vi "FTT Sreen.vi"(8 "error in (no error)":errorcluster caption="错误输入（无错误）", 11 "Main":T2={"Tite"="", "Base path"=path "", "Table"=[], "Stations"=[], "Shield Array"=[], "UPHs"=[], "VISA"={"VISA"="", "baud rate"=9600, "data bits"=8, "parity"=enum."None", "stop bits"=10, "flow control"=0}, "Path"={"roof"=path "", "Config"=path "", "Png"=path ""}, "Ctr"={"DB Dispaly"=refnum, "Error Table"=refnum, "Display"=refnum, "Login"=refnum, "Exit"=refnum, "FTT_Submit"=refnum}, "Login"={"User"="", "Grade"=""}, "information"={"cause"="", "Type"=enum."Inform", "code"=0, "Suroce"="", "Status"=FALSE}, "Local DB"={"Connstr"="", "Database"={"Constr"={"Driver"="", "Server"="", "User"="", "Pwd"="", "Database"=""}, "conn ref"=refnum, "State"=FALSE}}, "Remote DB"={"Connstr"="", "Database"={"Constr"={"Driver"="", "Server"="", "User"="", "Pwd"="", "Database"=""}, "conn ref"=refnum, "State"=FALSE}}, "FTT TV"="", "ExchangeTime"=0, "NVH"="", "EOL Path"=path ""} {"VISA"."flow control" items=["None", "XON/XOFF", "RTS/CTS", "XON/XOFF & RTS/CTS", "DTR/DSR", "XON/XOFF & DTR/DSR"]; "VISA"."stop bits" items=["1.0"=10, "1.5"=15, "2.0"=20]}) -> (0 "error out":errorcluster)   [LabVIEW 2014]
uses:
  Type'def/CN Product1_5 Ctr.ctl
  Type'def/CN Product1_4 Ctr.ctl
  Type'def/CN Product Ctr.ctl
  Type'def/Tab.ctl
  Type'def/MainCtr.ctl
  Type'def/UPH Config.ctl
  SubVI's/VISA/Ctr/VISA Ctr.ctl
  Type'def/Main Ctr Ref.ctl
  Type'def/User Login.ctl
  SubVI's/Database/Ctr/Conneect State.ctl
  SubVI's/Database/Ctr/Constr.ctl
  <vilib>/addons/database/Connection.llb/Conn ObjectReference.ctl
  Type'def/CN image Ctr.ctl
  <vilib>/picture/picture.llb/imagedata.ctl
  Type'def/CN Config Ctr.ctl
  <vilib>/addons/database/NI_Database_API.lvlib
panel:
  out "Tab":T1(array[ring])
  out "size(s)":i32
  out "Value":string
  out "Repaired":string
  out "Slash 04":string
  out "End?":bool
  out "Show Tab":T10
  out "Tab CN":enum32{"1/2", "1/3", "1/4", "1/5", "2/5", "3/5"}(tab)
  out "CN image2/2":T11
  out "CN image1/2":T11
  out "CN image3/3":T11
  out "CN image2/3":T11
  out "CN image1/3":T11
  out "CN image4/4":T12
  out "CN image3/4":T12
  out "CN image2/4":T12
  out "CN image1/4":T12
  out "CN image5/5":T13
  out "CN image4/5":T13
  out "CN image3/5":T13
  out "CN image2/5":T13
  out "CN image1/5":T13
  out "CN image5/6":T13
  out "CN image4/6":T13
  out "CN image3/6":T13
  out "CN image2/6":T13
  out "CN image1/6":T13
  out "CN image5/7":T13
  out "CN image4/7":T13
  out "CN image3/7":T13
  out "CN image2/7":T13
  out "CN image1/7":T13
  out "Roof Picture":picture
  out "Vehicle Picture":picture
  out "Line status":string
  out "UPH status":string
  out "Rollo Color status":string
  out "Model":string
  out "Slash 03":string
  out "Slash 01":string
  out "Slash 02":string
  out "FTT Rate":string
  out "Reject":string
  out "Target(%)":string
  out "Target now":string
  out "FTT":string
  out "Actual":string
  out "Plan":string
  out "Repaired and Reject Title":string
  out "Target and Actual Title":string
  out "FTT and FTT Rate Title":string
  out "Plan and Rate Title":string
  out "Error Info 3":string
  out "Error Info 2":string
  out "Error Info":string
  out "Error BG":u32(colorbox)
  out "Time":string
  out "Date":string
  out "Title":string
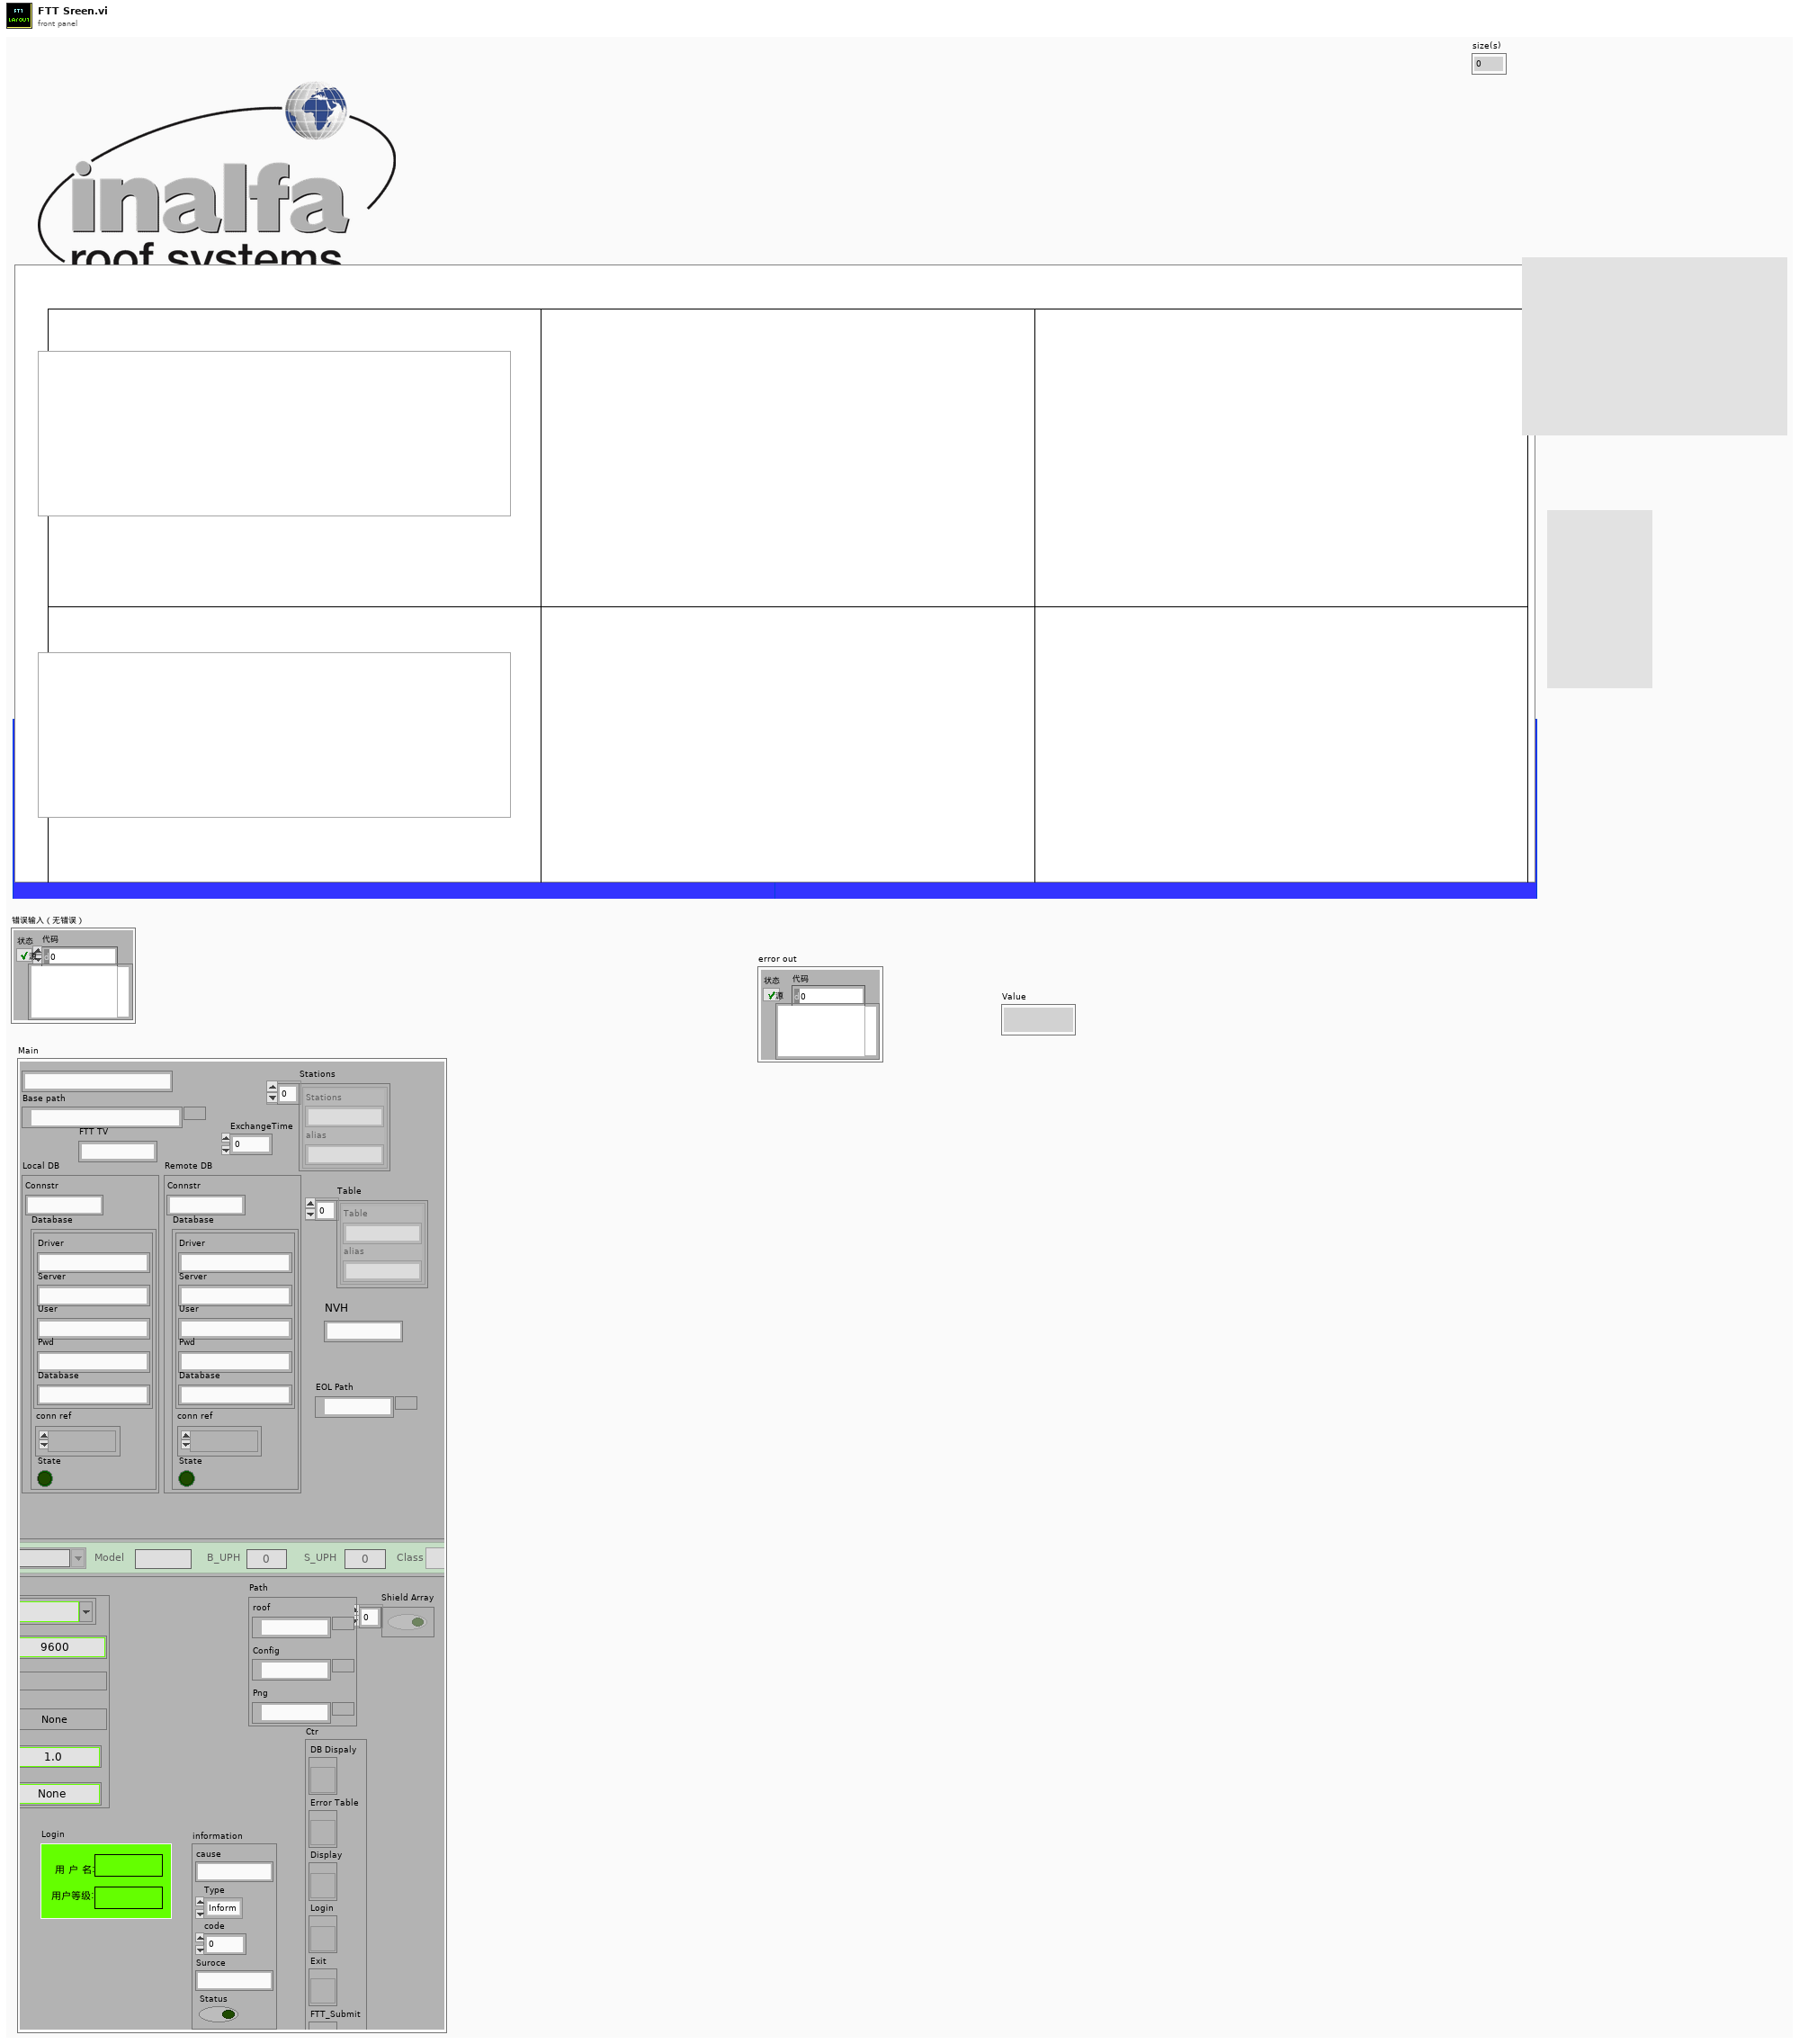
[diagram p1: front panel]
types:
  T1 = enum32{"1/2", "1/3", "1/4", "1/5", "2/5", "3/5"}[]
  T2 = typedef "MainCtr.ctl" = cluster{"Tite":string, "Base path":path, "Table":cluster{"Table":string, "alias":string}[], "Stations":cluster{"Stations":string, "alias":string}[], "Shield Array":bool[], "UPHs":T3[], "VISA":T4, "Path":cluster{"roof":path, "Config":path, "Png":path}, "Ctr":T5, "Login":T6, "information":cluster{"cause":string, "Type":enum16{"Inform", "Warning", "Alarm"}, "code":i32, "Suroce":string, "Status":bool}, "Local DB":cluster{"Connstr":string, "Database":T7}, "Remote DB":cluster{"Connstr":string, "Database":T7}, "FTT TV":string, "ExchangeTime":i32, "NVH":string, "EOL Path":path}
  T3 = typedef "UPH Config.ctl" = cluster{"Line_No":string, "Model":string, "B_UPH ":i16, "S_UPH  ":i16, "Class":enum16{"Big", "Small"}}
  T4 = typedef "VISA Ctr.ctl" = cluster{"VISA":refnum<visa-resource-name>, "baud rate":u32, "data bits":u16, "parity":enum16{"None", "Odd", "Even", "Mark", "Space"}, "stop bits":u16, "flow control":u16}
  T5 = typedef "Main Ctr Ref.ctl" = cluster{"DB Dispaly":refnum<vi>, "Error Table":refnum<vi>, "Display":refnum<vi>, "Login":refnum<vi>, "Exit":refnum<vi>, "FTT_Submit":refnum<vi>}
  T6 = typedef "User Login.ctl" = cluster{"User":string, "Grade":string}
  T7 = typedef "Conneect State.ctl" = cluster{"Constr":T8, "conn ref":T9, "State":bool}
  T8 = typedef "Constr.ctl" = cluster{"Driver":string, "Server":string, "User":string, "Pwd":string, "Database":string}
  T9 = typedef "NI_Database_API.lvlib/Conn ObjectReference.ctl" = refnum<k1>
  T10 = typedef "Tab.ctl" = enum32{"Customer and Shift Info", "Manufacture Info", "Device error info"}
  T11 = typedef "CN Product Ctr.ctl" = cluster{"2D Picture 3":picture, "Model":string, "Brand":string}
  T12 = typedef "CN Product1_4 Ctr.ctl" = cluster{"2D Picture 3":picture, "Model":string, "Brand":string}
  T13 = typedef "CN Product1_5 Ctr.ctl" = cluster{"2D Picture 3":picture, "Model":string, "Brand":string}
  T14 = typedef "imagedata.ctl" = cluster{"image type":i32, "image depth":i32, "image":u8[], "mask":u8[], "colors":u32[], "Rectangle":cluster{"left":i16, "top":i16, "right":i16, "bottom":i16}}
  T15 = cluster{"FTTColor":cluster{"Low":u32, "Middle":u32, "High":u32}, "TargetColor":cluster{"Low":u32, "Middle":u32, "High":u32}}
  T16 = cluster{"FTTRate":cluster{"Low":u32, "High":u32}, "TargetRate":cluster{"Low":u32, "High":u32}}
  T17 = typedef "CN image Ctr.ctl" = cluster{"Images":T14[], "filenames":string[], "Fit Zoom":dbl[], "CN Config":T18[], "CN Enable":T18[], "image Enable":T14[], "CN Ref Enable":refnum<vi>[], "Tab ":enum32{"1/2", "1/3", "1/4", "1/5", "2/5", "3/5"}[], "Pic Enable":refnum<vi>[]}
  T18 = typedef "CN Config Ctr.ctl" = cluster{"Model":string, "Pic_Name":string, "CarName":string, "En/Disable":bool}
  T19 = cluster{"Path":cluster{"roof":path, "Config":path, "Png":path}, "Exit":refnum<vi>, "Show Tab":refnum<vi>, "Target(%)":refnum<vi>, "Repaired":refnum<vi>, "Reject":refnum<vi>, "FTT":refnum<vi>, "FTT Rate":refnum<vi>, "Line status":refnum<vi>, "Vehicle Picture":refnum<vi>, "Roof Picture":refnum<vi>, "Time":refnum<vi>, "Date":refnum<vi>, "Title":refnum<vi>, "Error Info":refnum<vi>, "UPH status":refnum<vi>, "Rollo Color status":refnum<vi>, "Plan":refnum<vi>, "Actual":refnum<vi>, "Repaired":refnum<vi>, "Target now":refnum<vi>, "Range":cluster{"FTTRate":cluster{"Low":u32, "High":u32}, "TargetRate":cluster{"Low":u32, "High":u32}}, "Color":cluster{"FTTColor":cluster{"Low":u32, "Middle":u32, "High":u32}, "TargetColor":cluster{"Low":u32, "Middle":u32, "High":u32}}, "Ctr Color":cluster{"Label":string, "Color":u32}[], "CN Ctr Ref":refnum<vi>[], "CN image":T17, "Tab CN":refnum<vi>}
  T20 = cluster{"seconds":dbl, "Pages":i32, "element":enum32{"1/2", "1/3", "1/4", "1/5", "2/5", "3/5"}}
  T21 = typedef "Main FTT.ctl" = cluster{"Line_Name":string, "Model":string, "Line_State":string, "Color":string, "UPH":string, "Plan":string, "Target Rate":string, "Target":string, "Actual":string, "FTT":string, "FTT Rate":string, "Repaired":string, "Reject":string}
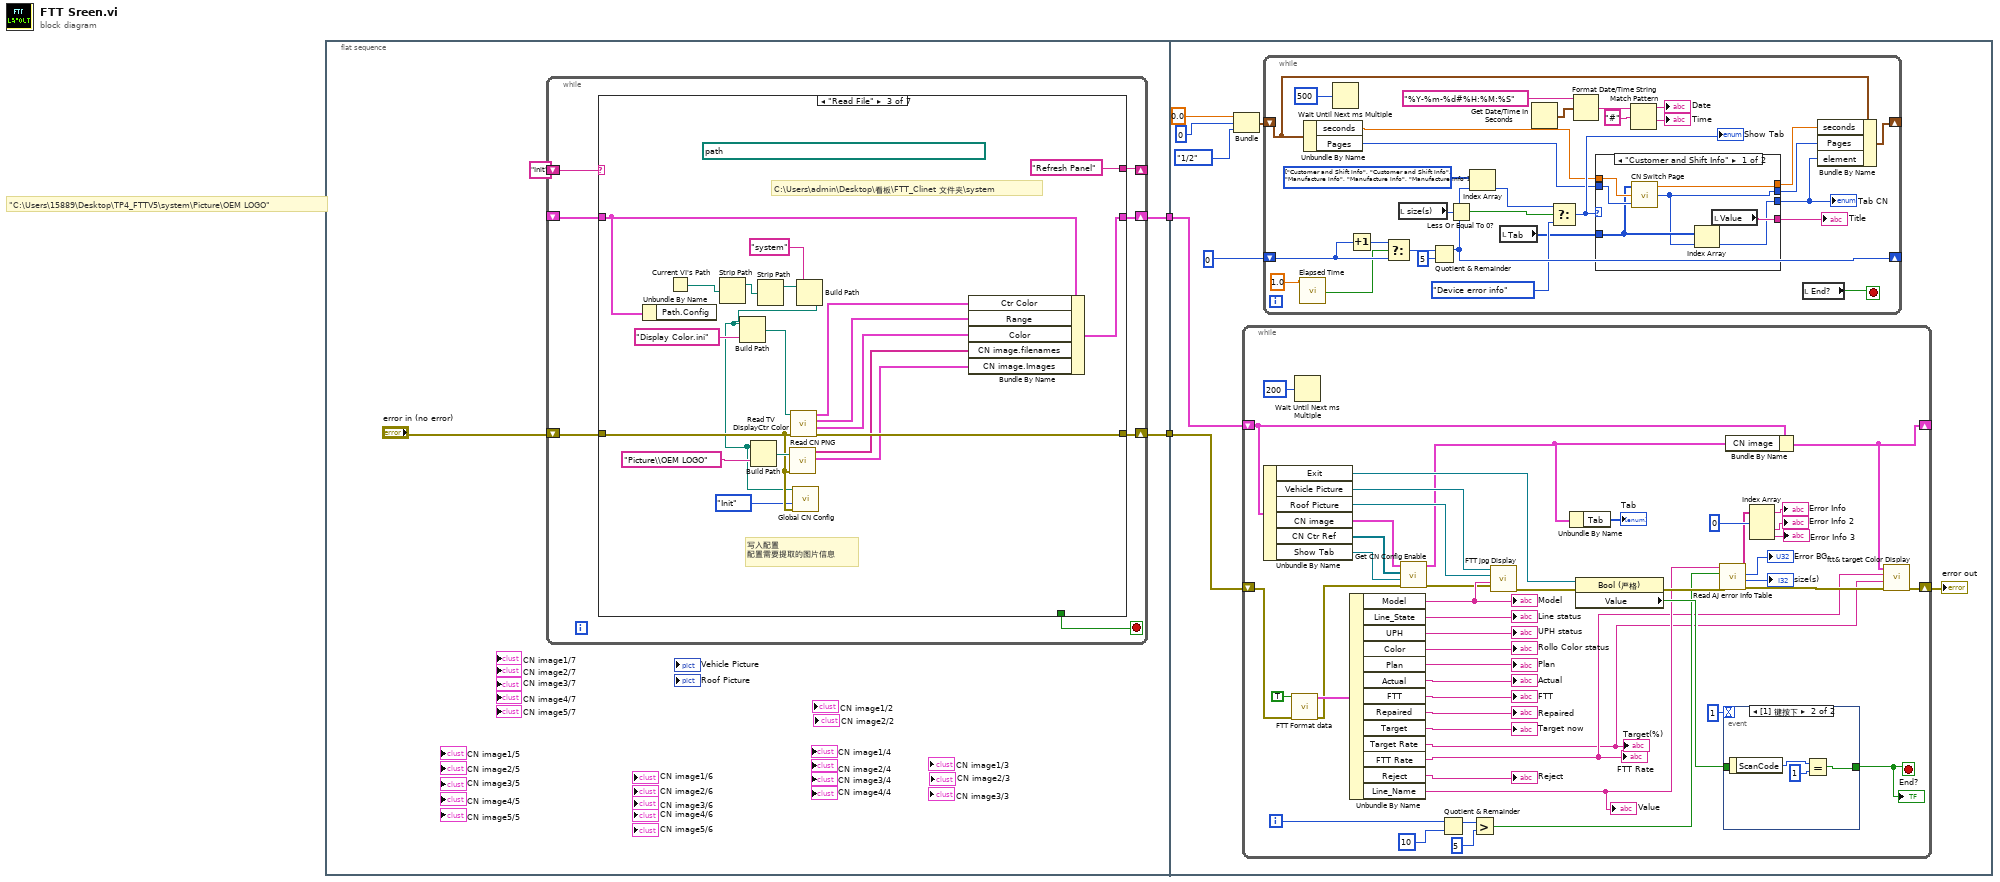
[diagram p0: block diagram]
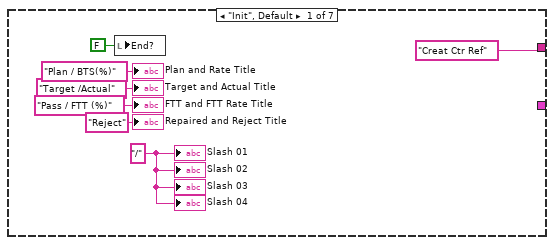
[diagram p2: hidden frame]
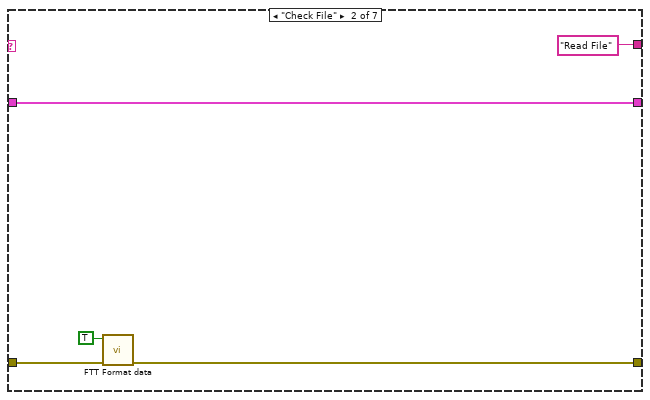
[diagram p3: hidden frame]
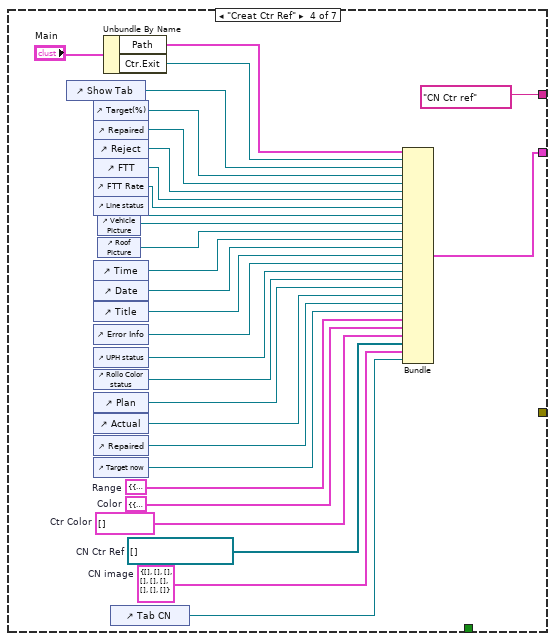
[diagram p4: hidden frame]
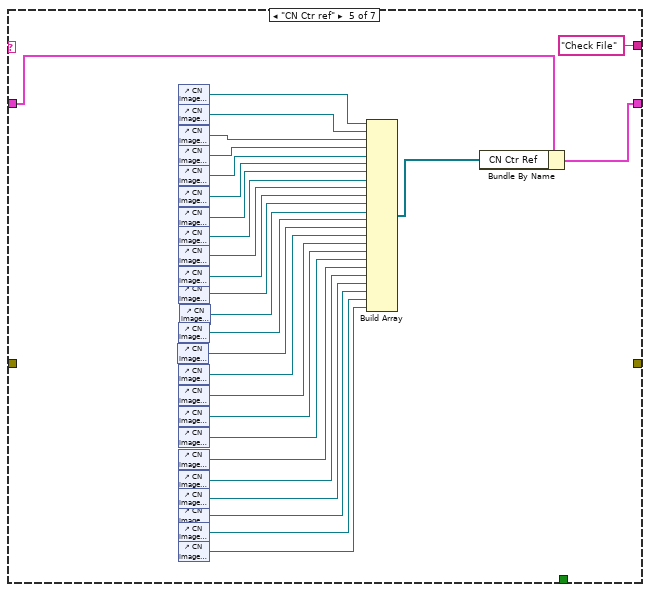
[diagram p5: hidden frame]
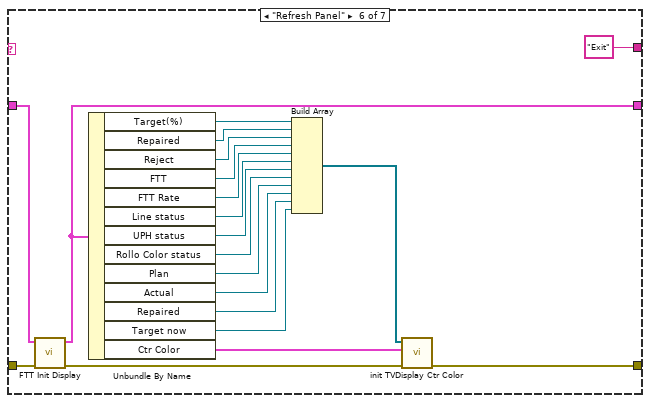
[diagram p6: hidden frame]
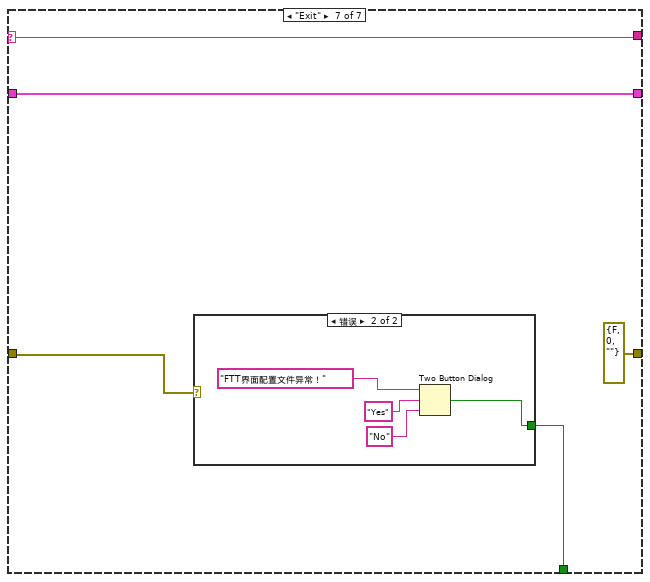
[diagram p7: hidden frame]
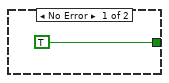
[diagram p8: hidden frame]
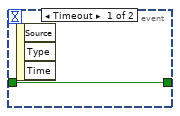
[diagram p9: hidden frame]
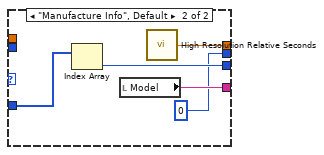
[diagram p10: hidden frame]
diagram:
  # "\"C:\\Users\\15889\\Desktop\\TP4_FTTV5\\system\\Picture\\OEM LOGO\""
  n1 = flat-sequence {
    tunnel: [w4] -> w2
    tunnel: [w3] -> w1
    tunnel: w2 -> [w140]
    tunnel: w1 -> [w141]
    frame #0 {
      n2 = while {
        shift-right: [w12] -> _
        shift-left: "Init" -> [w13]
        shift-right: [w10] -> w3
        shift-left: _ -> [w9]
        shift-right: [w7] -> w4
        shift-left: "error in (no error)" -> [w8]
        stop <- w11 stop-if-true
        n3 = case shown="\"Read File\"" w13 {
          selector: w13 -> [_ _ _ _ _ _ w127]
          tunnel: ["Creat Ctr Ref" "Read File" "Refresh Panel" "CN Ctr ref" "Check File" "Exit" w127] -> w12
          tunnel: [_ _ _ _ _ _ w124] -> w11
          tunnel: [_ w24 w40 w63 w102 w104 w128] -> w10
          tunnel: w9 -> [_ w24 w41 _ w103 w105 w128]
          tunnel: w8 -> [_ w23 w32 _ _ w122 w125]
          tunnel: [_ w22 w42 _ _ w106 errorcluster {"status"=FALSE, "code"=0, "source"=""} ("error out")] -> w7
          frame "Init", Default {
            w16 = "/" ("Slash 01")
            n4 = local write "End?"(FALSE ("End?")) -> ()
            "FTT and FTT Rate Title" <- "Pass / FTT (%)" ("FTT Title")
            "Plan and Rate Title" <- "Plan / BTS(%)" ("Target and Color Title")
            "Target and Actual Title" <- "Target /Actual" ("FTT Title 3")
            "Repaired and Reject Title" <- "Reject" ("FTT Title 4")
            "Slash 02" <- w16
            "Slash 01" <- w16
            "Slash 03" <- w16
            "Slash 04" <- w16
          }
          frame "Check File" {
            n5 = call "FTT Format data.vi"("error in (no error)"=w23, "W/R"=TRUE) -> ("error out"=w22:errorcluster)  [unwired: 6 in, 3 out]
          }
          frame "Read File" {
            (unwired) path "C:/Users/admin/Desktop/V254/FTT Sreen 文件夹/system" ("Path.Config")
            # "写入配置\n配置需要提取的图片信息"
            # "C:\\Users\\admin\\Desktop\\看板\\FTT_Clinet 文件夹\\system"
            n6 = Unbundle By Name(w41) -> ()  [unwired: 1 out]
            n7 = Current VI's Path() -> (path=w30:path)
            n8 = Strip Path(path=w30) -> (stripped path=w29:path)  [unwired: 1 out]
            n9 = Strip Path(path=w29) -> (stripped path=w28:path)  [unwired: 1 out]
            n10 = Build Path(base path=w28, name or relative path="system" ("名称或相对路径")) -> (appended path=w26:path)
            n11 = Build Path(base path=w26, name or relative path="Display Color.ini") -> (appended path=w43:path)
            n12 = Build Path(base path=w26, name or relative path="Picture\\OEM LOGO") -> (appended path=w36:path)
            n13 = call "Read CN PNG.vi"("error in (no error)"=w32, "floder Path"=w36) -> ("Images"=w33:T14[], "filenames"=w34:string[])  [unwired: 7 in, 1 out]
            n14 = call "Read TV DisplayCtr Color.vi"("error in (no error)"=w32, "Path"=w43) -> ("error out"=w42:errorcluster, "Color"=w37:T15, "Range"=w38:T16, "Array"=w39:cluster{"Label":string, "Color":u32}[])  [unwired: 6 in]
            n15 = call "Global CN Config.vi"("error in (no error)"=w32, "Mode"=enum16{"Init", "Read", "Write"}."Init", "Path"=w26) -> ()  [unwired: 7 in, 2 out]
            n16 = Bundle By Name(cluster=w41, "Ctr Color"=w39, "Range"=w38, "Color"=w37, "CN image.filenames"=w34, "CN image.Images"=w33) -> (w40:T19)
          }
          frame "Creat Ctr Ref" {
            w47 = T17 {"Images"=[], "filenames"=[], "Fit Zoom"=[], "CN Config"=[], "CN Enable"=[], "image Enable"=[], "CN Ref Enable"=[], "Tab "=[], "Pic Enable"=[]}  # CN image
            w48 = refnum<vi>[] []  # CN Ctr Ref
            w51 = cluster{"Label":string, "Color":u32}[] []  # Ctr Color
            w52 = T15 {"FTTColor"={"Low"=0, "Middle"=0, "High"=0}, "TargetColor"={"Low"=0, "Middle"=0, "High"=0}}  # Color
            w53 = T16 {"FTTRate"={"Low"=0, "High"=0}, "TargetRate"={"Low"=0, "High"=0}}  # Range
            n17 = control-ref of="Show Tab"() -> (w75:refnum<vi>)
            n18 = control-ref of="Target(%)"() -> (w74:refnum<vi>)
            n19 = control-ref of="Repaired"() -> (w73:refnum<vi>)
            n20 = control-ref of="Reject"() -> (w72:refnum<vi>)
            n21 = control-ref of="FTT"() -> (w71:refnum<vi>)
            n22 = control-ref of="FTT Rate"() -> (w70:refnum<vi>)
            n23 = control-ref of="Line status"() -> (w69:refnum<vi>)
            n24 = control-ref of="Time"() -> (w66:refnum<vi>)
            n25 = control-ref of="Date"() -> (w65:refnum<vi>)
            n26 = control-ref of="Title"() -> (w64:refnum<vi>)
            n27 = control-ref of="Error Info"() -> (w60:refnum<vi>)
            n28 = control-ref of="UPH status"() -> (w59:refnum<vi>)
            n29 = control-ref of="Rollo Color status"() -> (w58:refnum<vi>)
            n30 = control-ref of="Plan"() -> (w57:refnum<vi>)
            n31 = control-ref of="Actual"() -> (w56:refnum<vi>)
            n32 = control-ref of="Repaired"() -> (w55:refnum<vi>)
            n33 = control-ref of="Target now"() -> (w54:refnum<vi>)
            n34 = control-ref of="Vehicle Picture"() -> (w68:refnum<vi>)
            n35 = control-ref of="Roof Picture"() -> (w67:refnum<vi>)
            n36 = Unbundle By Name("Main") -> ("Path"=w49:cluster{"roof":path, "Config":path, "Png":path}, "Ctr.Exit"=w61:refnum<vi>)
            n37 = control-ref of="Tab CN"() -> (w46:refnum<vi>)
            n38 = Bundle("Path"=w49, "Exit"=w61, "Show Tab"=w75, "Target(%)"=w74, "Repaired"=w73, "Reject"=w72, "FTT"=w71, "FTT Rate"=w70, "Line status"=w69, "Vehicle Picture"=w68, "Roof Picture"=w67, "Time"=w66, "Date"=w65, "Title"=w64, "Error Info"=w60, "UPH status"=w59, "Rollo Color status"=w58, "Plan"=w57, "Actual"=w56, "Repaired"=w55, "Target now"=w54, "Range"=w53, "Color"=w52, "Ctr Color"=w51, "CN Ctr Ref"=w48, "CN image"=w47, "Tab CN"=w46) -> (w63:T19)  [unwired: 1 in]
          }
          frame "CN Ctr ref" {
            n39 = control-ref of="CN image5/5"() -> (w88:refnum<vi>)
            n40 = control-ref of="CN image1/2"() -> (w101:refnum<vi>)
            n41 = control-ref of="CN image2/2"() -> (w100:refnum<vi>)
            n42 = control-ref of="CN image1/3"() -> (w99:refnum<vi>)
            n43 = control-ref of="CN image2/3"() -> (w98:refnum<vi>)
            n44 = control-ref of="CN image3/3"() -> (w97:refnum<vi>)
            n45 = control-ref of="CN image1/4"() -> (w96:refnum<vi>)
            n46 = control-ref of="CN image2/4"() -> (w95:refnum<vi>)
            n47 = control-ref of="CN image3/4"() -> (w94:refnum<vi>)
            n48 = control-ref of="CN image4/4"() -> (w93:refnum<vi>)
            n49 = control-ref of="CN image1/5"() -> (w92:refnum<vi>)
            n50 = control-ref of="CN image2/5"() -> (w91:refnum<vi>)
            n51 = control-ref of="CN image4/5"() -> (w89:refnum<vi>)
            n52 = control-ref of="CN image1/6"() -> (w87:refnum<vi>)
            n53 = control-ref of="CN image2/6"() -> (w86:refnum<vi>)
            n54 = control-ref of="CN image3/6"() -> (w85:refnum<vi>)
            n55 = control-ref of="CN image4/6"() -> (w84:refnum<vi>)
            n56 = control-ref of="CN image5/6"() -> (w83:refnum<vi>)
            n57 = control-ref of="CN image1/7"() -> (w82:refnum<vi>)
            n58 = control-ref of="CN image2/7"() -> (w81:refnum<vi>)
            n59 = control-ref of="CN image3/7"() -> (w80:refnum<vi>)
            n60 = control-ref of="CN image4/7"() -> (w79:refnum<vi>)
            n61 = control-ref of="CN image5/7"() -> (w78:refnum<vi>)
            n62 = control-ref of="CN image3/5"() -> (w90:refnum<vi>)
            n63 = Build Array(w101, w100, w99, w98, w97, w96, w95, w94, w93, w92, w91, w90, w89, w88, w87, w86, w85, w84, w83, w82, w81, w80, w79, w78) -> (w77:refnum<vi>[])
            n64 = Bundle By Name(cluster=w103, "CN Ctr Ref"=w77) -> (w102:T19)
          }
          frame "Refresh Panel" {
            n65 = call "FTT Init Display.vi"("error in (no error)"=w122, "Cluster 2"=w105) -> ("error out"=w109:errorcluster, "Cluster out"=w104:T19)  [unwired: 8 in]
            n66 = Unbundle By Name(w104) -> ("Target(%)"=w121:refnum<vi>, "Repaired"=w120:refnum<vi>, "Reject"=w119:refnum<vi>, "FTT"=w118:refnum<vi>, "FTT Rate"=w117:refnum<vi>, "Line status"=w116:refnum<vi>, "UPH status"=w115:refnum<vi>, "Rollo Color status"=w114:refnum<vi>, "Plan"=w113:refnum<vi>, "Actual"=w112:refnum<vi>, "Repaired"=w111:refnum<vi>, "Target now"=w110:refnum<vi>, "Ctr Color"=w107:cluster{"Label":string, "Color":u32}[])
            n67 = Build Array(w121, w120, w119, w118, w117, w116, w115, w114, w113, w112, w111, w110) -> (w108:refnum<vi>[])
            n68 = call "init TVDisplay Ctr Color.vi"("error in (no error)"=w109, "Ctr Color"=w107, "appended array"=w108) -> ("error out"=w106:errorcluster)  [unwired: 8 in]
          }
          frame "Exit" {
            n69 = case shown="错误" w125 {
              tunnel: [TRUE w130] -> w124
              frame No Error {
              }
              frame Error {
                n70 = Two Button Dialog(message="FTT界面配置文件异常！" ("消息"), 1:"No" ("F按钮名称（“取消”）"), 2:"Yes" ("T按钮名称（“确定”）")) -> (T button?=w130:bool)
              }
            }
          }
        }
      }
    }
    frame #1 {
      n71 = Bundle("seconds"=0.0, "Pages"=0, "element"=enum32{"1/2", "1/3", "1/4", "1/5", "2/5", "3/5"}."1/2") -> (w134:T20)  [unwired: 1 in]
      n72 = while {
        shift-right: [w153] -> w139
        shift-left: w140 -> [w181]
        shift-right: [w144] -> _
        shift-left: w141 -> [w147]
        i -> [w167]
        stop <- w169 stop-if-true
        n73 = Unbundle By Name(w147) -> ("Exit"=w171:refnum<vi>, "Vehicle Picture"=w188:refnum<vi>, "Roof Picture"=w187:refnum<vi>, "CN image"=w150:T17, "CN Ctr Ref"=w146:refnum<vi>[], "Show Tab"=w145:refnum<vi>)
        n74 = call "FTT Format data.vi"("error in (no error)"=w181, "W/R"=TRUE) -> ("error out"=w149:errorcluster, "Display"=w186:T21)  [unwired: 6 in, 2 out]
        n75 = Wait Until Next ms Multiple(millisecond multiple=u32 200) -> ()  [unwired: 1 out]
        n76 = Unbundle By Name(w186) -> ("Model"=w184:string, "Line_State"=→"Line status":string, "UPH"=→"UPH status":string, "Color"=→"Rollo Color status":string, "Plan"=→"Plan":string, "Actual"=→"Actual":string, "FTT"=→"FTT":string, "Repaired"=→"Repaired":string, "Target"=→"Target now":string, "Target Rate"=w151:string, "FTT Rate"=w152:string, "Reject"=→"Reject":string, "Line_Name"=w155:string)
        "Model" <- w184
        "Target(%)" <- w151
        "FTT Rate" <- w152
        "Value" <- w155
        n77 = call "Get CN Config Enable.vi"("error in (no error)"=w149, "Show Tab"=w145, "CN Pic Ref"=w146, "CN image"=w150) -> ("error out"=w148:errorcluster, "CN image out"=w143:T17)  [unwired: 6 in]
        n78 = Quotient & Remainder(x=w167, y=10) -> (x-y*floor(x/y)=w165:i32)  [unwired: 1 out]
        n79 = Greater?(x=w165, y=5) -> (0:w163:bool)
        n80 = call "FTT jpg Display.vi"("error in (no error)"=w148, "Model"=w184, "Roof Picture"=w187, "Vehicle Picture"=w188) -> ("错误输出"=w172:errorcluster)  [unwired: 7 in]
        n81 = Unbundle By Name(w143) -> ("Tab"=→"Tab":T1)
        n82 = property class="Bool (严格)"(reference=w171, error in=w172) -> (error out=w168:errorcluster, "Value"=w170:bool)  [unwired: 1 out]
        n83 = call "Read AJ error Info Table.vi"("error in (no error)"=w168, "s"=w163, "Linename"=w155) -> ("error IO"=w154:errorcluster, "size(s)"=→"size(s)":i32, "Error BG"=→"Error BG":u32, "Array"=w156:string[])  [unwired: 5 in]
        n84 = event shown="[1] 键按下" {
          selector: _ -> [_ _]
          dyn-events: _ -> [_ _]
          timeout: 1 -> [_ _]
          tunnel: [w190 w191] -> w169
          tunnel: w170 -> [w190 _]
          event Timeout {
            n85 = event-data() -> ()  [unwired: 1 in, 3 out]
          }
          event Key Down {
            n86 = event-data() -> ("ScanCode"=w193:i16)  [unwired: 1 in]
            n87 = Equal?(x=w193, y=i16 1) -> (x = y?=w191:bool)
          }
        }
        "End?" <- w169
        n88 = Bundle By Name(cluster=w147, "CN image"=w143) -> (w144:T19)
        n89 = Index Array(array=w156, index #1=0 ("index")) -> (element #1=→"Error Info":string, element #2=→"Error Info 2":string, element #3=→"Error Info 3":string)  [unwired: 2 in]
        n90 = call "ftt& target Color Display.vi"("error in (no error)"=w154, "Tatget"=w151, "ftt"=w152, "Cluster"=w144) -> ("error out"=w153:errorcluster)  [unwired: 7 in]
      }
      "error out" <- w139
      n91 = while {
        shift-right: [w212] -> _
        shift-left: u64 0 -> [w221]
        shift-right: [w199] -> _
        shift-left: w134 -> [w200]
        stop <- w208 stop-if-true
        w219 = T10[] [enum."Customer and Shift Info", enum."Customer and Shift Info", enum."Manufacture Info", enum."Manufacture Info", enum."Manufacture Info"] items=["Customer and Shift Info", "Manufacture Info", "Device error info"]
        n92 = call "Elapsed Time"("Time Target (s)"=1.0) -> ("Time has Elapsed"=w207:bool)  [unwired: 11 in, 7 out]
        n93 = Unbundle By Name(w200) -> ("seconds"=w195:dbl, "Pages"=w194:i32)
        n94 = Wait Until Next ms Multiple(millisecond multiple=u32 500) -> ()  [unwired: 1 out]
        n95 = Increment(x=w221) -> (x+1=w220:u64)
        n96 = Select(t=w220, s=w207, f=w221) -> (s? t:f=w214:u64)
        n97 = local read "size(s)"() -> (w203:i32)
        n98 = Quotient & Remainder(x=w214, y=u64 5) -> (x-y*floor(x/y)=w212:u64)  [unwired: 1 out]
        n99 = Less Or Equal To 0?(x=w203) -> (x <= 0?=w202:bool)
        n100 = Index Array(array=w219, index=w212) -> (element=w205:T10)
        n101 = local read "Tab"() -> (w201:T1)
        n102 = Get Date/Time In Seconds() -> (seconds since 1Jan1904=w215:timestamp)
        n103 = Select(t=w205, s=w202, f=Tab."Device error info" ("element")) -> (s? t:f=w204:T10)
        "Show Tab" <- w204
        n104 = Format Date/Time String(time format string (%c)="%Y-%m-%d#%H:%M:%S", seconds (now)=w215) -> (date/time string=w216:string)  [unwired: 1 in]
        n105 = case shown="\"Customer and Shift Info\"" w204 {
          tunnel: [w230 w235] -> w211
          tunnel: w201 -> [w226 w234]
          tunnel: [w224 w233] -> w196
          tunnel: [w227 w232] -> w198
          tunnel: [w225 0] -> w197
          tunnel: w195 -> [w229 _]
          tunnel: w194 -> [w228 _]
          frame "Customer and Shift Info" {
            n106 = call "CN Switch Page.vi"("Page"=w228, "Scond"=w229, "Tab"=w226) -> ("Page"=w225:i32, "scond"=w227:dbl)  [unwired: 1 out]
            n107 = Index Array(array=w226, index=w225) -> (element=w224:enum32{"1/2", "1/3", "1/4", "1/5", "2/5", "3/5"})
            n108 = local read "Value"() -> (w230:string)
          }
          frame "Manufacture Info", Default {
            n109 = Index Array(array=w234) -> (element=w233:enum32{"1/2", "1/3", "1/4", "1/5", "2/5", "3/5"})  [unwired: 1 in]
            n110 = local read "Model"() -> (w235:string)
            n111 = call <vilib>:"High Resolution Relative Seconds.vi"() -> ("relative seconds"=w232:dbl)
          }
        }
        "Title" <- w211
        "Tab CN" <- w196
        n112 = Match Pattern(string=w216, regular expression="#") -> (before substring=→"Date":string, after substring=→"Time":string)  [unwired: 1 in, 2 out]
        n113 = local read "End?"() -> (w208:bool)
        n114 = Bundle By Name(cluster=w200, "seconds"=w198, "Pages"=w197, "element"=w196) -> (w199:T20)
      }
    }
  }
